vi "min_jerk_params.vi"(1 "Action (Read)":T9=enum."Read", 4 "ETH Mike Model":T8) -> (16 "PID Settings":T1={"Gains"={"K(e)"=0.006, "Kp"=0.8, "Ki"=6.0, "Kd"=0.003}, "Non-linear gain"={"Non-linear gain P"=enum."exponential", "Non-linear gain I"=enum."off", "Non-linear gain D"=enum."off"}, "D-Part variable"=enum."process variable", "Velocity estimate dy/dt"=enum."external", "Anti reset windup"=TRUE, "I-Part error band"=inf, "Output range"={"output high"=0.0, "output low"=0.0}})   [LabVIEW 2019]
uses:
  ReadOnlyGlobalActions.ctl
  ETHMikeModel.ctl
  ENPID/PID_Settings.ctl
  ENPID/Gains.ctl
  ENPID/NonLinearGainParams.ctl
  ENPID/NonLinearGain.ctl
  ENPID/DPartVariable.ctl
  ENPID/VelocityEstimate.ctl
  ENPID/OutputRange.ctl
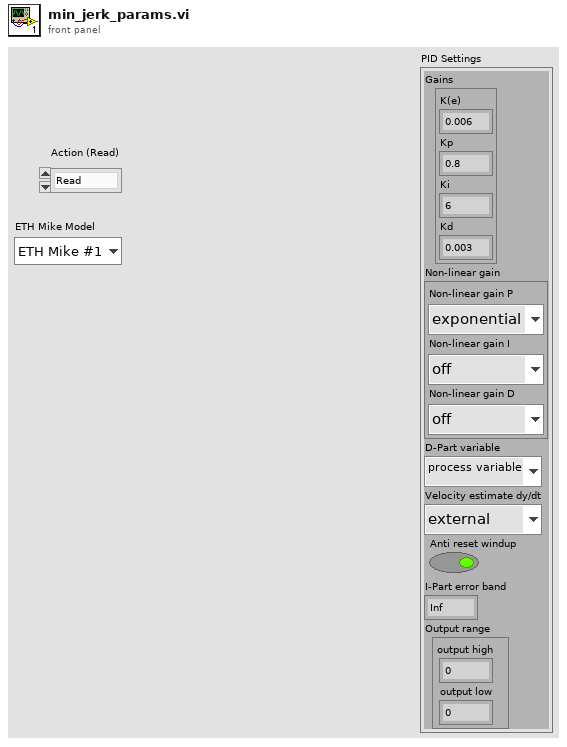
[diagram p1: front panel]
types:
  T1 = typedef "PID_Settings.ctl" = cluster{"Gains":T2, "Non-linear gain":T3, "D-Part variable":T5, "Velocity estimate dy/dt":T6, "Anti reset windup":bool, "I-Part error band":dbl, "Output range":T7}
  T2 = typedef "Gains.ctl" = cluster{"K(e)":dbl, "Kp":dbl, "Ki":dbl, "Kd":dbl}
  T3 = typedef "NonLinearGainParams.ctl" = cluster{"Non-linear gain P":T4, "Non-linear gain I":T4, "Non-linear gain D":T4}
  T4 = typedef "NonLinearGain.ctl" = enum16{"exponential", "quadratic", "off"}
  T5 = typedef "DPartVariable.ctl" = enum16{"error", "process variable"}
  T6 = typedef "VelocityEstimate.ctl" = enum16{"derivative", "external"}
  T7 = typedef "OutputRange.ctl" = cluster{"output high":dbl, "output low":dbl}
  T8 = typedef "ETHMikeModel.ctl" = enum16{"ETH Mike #1", "ETH Mike #2", "ETH Mike #3", "ETH Mike #4", "ETH MIKE #5", "ETH Mike #6"}
  T9 = typedef "ReadOnlyGlobalActions.ctl" = enum16{"Initialize", "Read", "Write"}
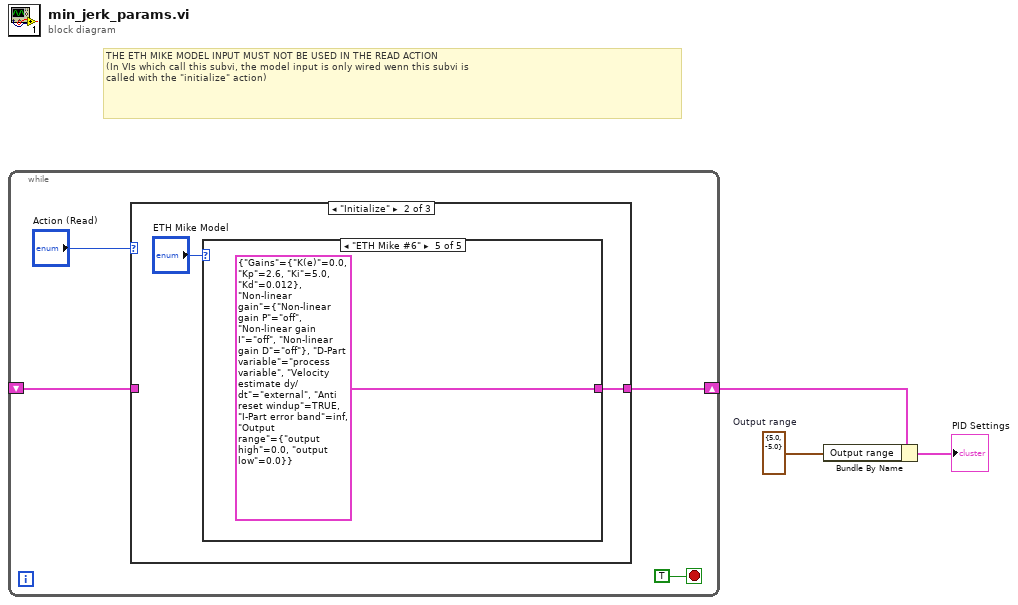
[diagram p0: block diagram]
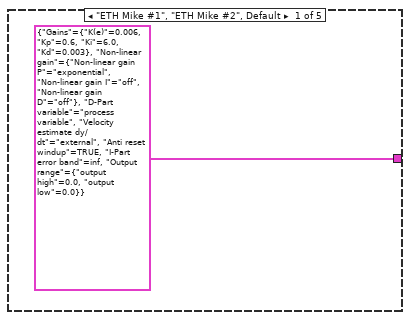
[diagram p3: hidden frame]
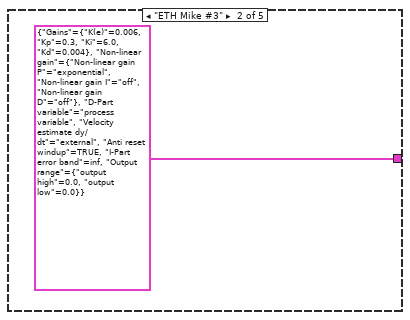
[diagram p4: hidden frame]
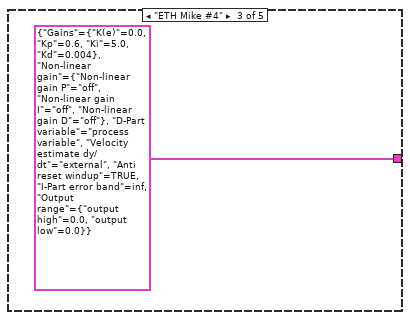
[diagram p5: hidden frame]
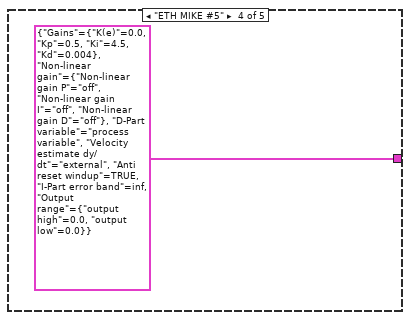
[diagram p6: hidden frame]
diagram:
  w1 = T7 {"output high"=5.0, "output low"=-5.0}  # Output range
  # "THE ETH MIKE MODEL INPUT MUST NOT BE USED IN THE READ ACTION\n(In VIs which call this subvi, the model input is only wired wenn this subvi is\ncalled with the \"initialize\" action)"
  n1 = while {
    shift-right: [w5] -> w2
    shift-left: _ -> [w4]
    stop <- TRUE stop-if-true
    n2 = case shown="\"Initialize\"" "Action (Read)" {
      tunnel: [w8 w9 w16] -> w5
      tunnel: w4 -> [w8 _ w16]
      frame "Read" {
      }
      frame "Initialize" {
        n3 = case shown="\"ETH Mike #6\"" "ETH Mike Model" {
          tunnel: [T1 {"Gains"={"K(e)"=0.006, "Kp"=0.6, "Ki"=6.0, "Kd"=0.003}, "Non-linear gain"={"Non-linear gain P"=enum."exponential", "Non-linear gain I"=enum."off", "Non-linear gain D"=enum."off"}, "D-Part variable"=enum."process variable", "Velocity estimate dy/dt"=enum."external", "Anti reset windup"=TRUE, "I-Part error band"=inf, "Output range"={"output high"=0.0, "output low"=0.0}} ("PID Settings") T1 {"Gains"={"K(e)"=0.006, "Kp"=0.3, "Ki"=6.0, "Kd"=0.004}, "Non-linear gain"={"Non-linear gain P"=enum."exponential", "Non-linear gain I"=enum."off", "Non-linear gain D"=enum."off"}, "D-Part variable"=enum."process variable", "Velocity estimate dy/dt"=enum."external", "Anti reset windup"=TRUE, "I-Part error band"=inf, "Output range"={"output high"=0.0, "output low"=0.0}} ("PID Settings") T1 {"Gains"={"K(e)"=0.0, "Kp"=0.6, "Ki"=5.0, "Kd"=0.004}, "Non-linear gain"={"Non-linear gain P"=enum."off", "Non-linear gain I"=enum."off", "Non-linear gain D"=enum."off"}, "D-Part variable"=enum."process variable", "Velocity estimate dy/dt"=enum."external", "Anti reset windup"=TRUE, "I-Part error band"=inf, "Output range"={"output high"=0.0, "output low"=0.0}} ("PID Settings") T1 {"Gains"={"K(e)"=0.0, "Kp"=0.5, "Ki"=4.5, "Kd"=0.004}, "Non-linear gain"={"Non-linear gain P"=enum."off", "Non-linear gain I"=enum."off", "Non-linear gain D"=enum."off"}, "D-Part variable"=enum."process variable", "Velocity estimate dy/dt"=enum."external", "Anti reset windup"=TRUE, "I-Part error band"=inf, "Output range"={"output high"=0.0, "output low"=0.0}} ("PID Settings") T1 {"Gains"={"K(e)"=0.0, "Kp"=2.6, "Ki"=5.0, "Kd"=0.012}, "Non-linear gain"={"Non-linear gain P"=enum."off", "Non-linear gain I"=enum."off", "Non-linear gain D"=enum."off"}, "D-Part variable"=enum."process variable", "Velocity estimate dy/dt"=enum."external", "Anti reset windup"=TRUE, "I-Part error band"=inf, "Output range"={"output high"=0.0, "output low"=0.0}} ("PID Settings")] -> w9
          frame "ETH Mike #1", "ETH Mike #2", Default {
          }
          frame "ETH Mike #3" {
          }
          frame "ETH Mike #4" {
          }
          frame "ETH MIKE #5" {
          }
          frame "ETH Mike #6" {
          }
        }
      }
      frame "Write" {
        # "Write action not supported"
      }
    }
  }
  n4 = Bundle By Name(cluster=w2, "Output range"=w1) -> (→"PID Settings":T1)
